vi "TestEnumerateCameraDevices.vi"(8 "error in (no error)":errorcluster, 11 "Test Case In":refnum<class "CameraManager.lvclass">) -> (0 "error out":errorcluster, 3 "Test Case Out":refnum<class "CameraManager.lvclass">)   [LabVIEW 2020, in "g_ar_toolkit.test.lvlib" / "CameraManager.lvclass"]
uses:
  CameraManager.lvclass
  C:/Program Files (x86)/National Instruments/LabVIEW 2020/vi.lib/Astemes/LUnit/Test Case.lvclass
  <vilib>/Astemes/LUnit/Test Case.lvclass/Test Case.ctl
  <vilib>/Astemes/LUnit/Append Fail Result.vi
  <vilib>/Astemes/LUnit/Append Pass Result.vi
  <vilib>/Astemes/LUnit/Run In UI.vi
  <vilib>/Utility/error.llb/Clear Errors.vi
  CameraManager.lvclass/CameraManager.ctl
  g_ar_toolkit.capture/g_ar_toolkit.capture.lvlib
  <vilib>/Astemes/LUnit/Test Case.lvclass
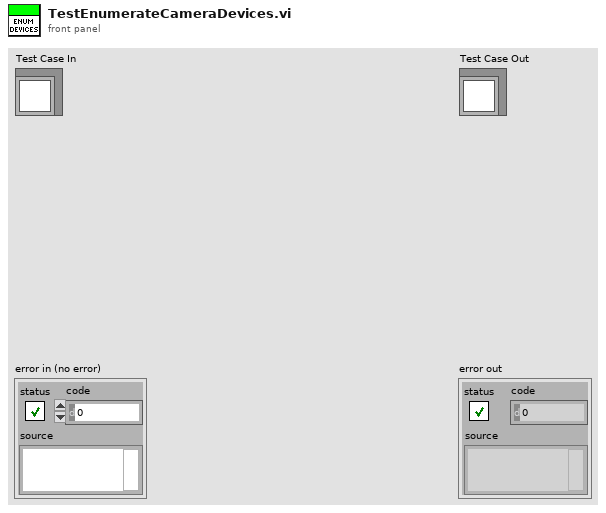
[diagram p1: front panel]
types:
  T1 = typedef "g_ar_toolkit.capture.lvlib/Stream.lvclass/Device Enumeration.ctl" = cluster{"Name":string, "Streams":set{T2}}
  T2 = typedef "g_ar_toolkit.capture.lvlib/Stream.lvclass/Stream Parameters.ctl" = cluster{"Width":u16, "Height":u16, "FPS":u8}
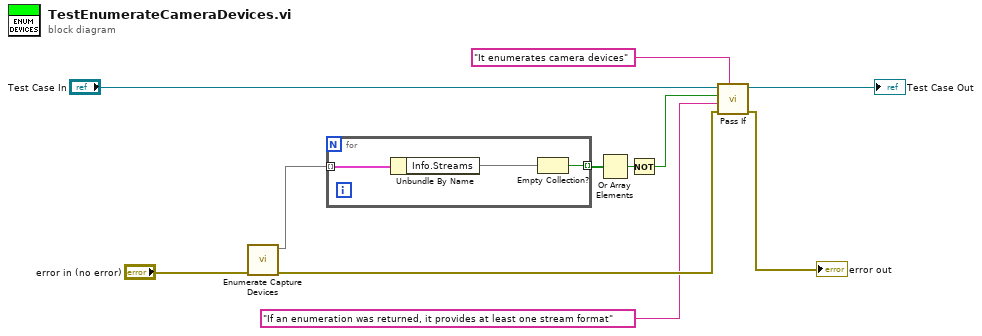
[diagram p0: block diagram]
diagram:
  n1 = call "Enumerate Capture Devices.vi"("error in (no error)"="error in (no error)") -> ("error out"=w7:errorcluster, "Devices"=w1:map{string, T1})  [unwired: 9 in]
  n2 = for {
    tunnel: w1 -> [w14] mode=indexing
    tunnel: [w12] -> w5 mode=indexing
    n3 = Unbundle By Name(w14) -> ("Info.Streams"=w13:set{T2})
    n4 = Empty Collection?(1:w13) -> (0:w12:bool)
  }
  n5 = Or Array Elements(Boolean array=w5) -> (logical OR=w4:bool)
  n6 = Not(x=w4) -> (.not. x?=w2:bool)
  n7 = call <vilib>:"Pass If.vi"("Description"="It enumerates camera devices", "error in (no error)"=w7, "Message"="If an enumeration was returned, it provides at least one stream format", "Pass?"=w2, "LUnit Test Case In"="Test Case In") -> ("error out"=→"error out":errorcluster, "LUnit Test Case Out"=→"Test Case Out":refnum<class "CameraManager.lvclass">)  [unwired: 5 in]
